vi "FFOvl.vi"(1 "Drv":u32=1) -> (0 "FFOvl":u8)   [LabVIEW 2017]
uses:
  ESLSCDLL.dll
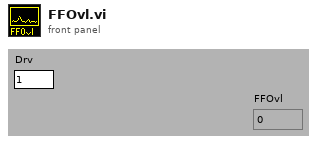
[diagram p1: front panel]
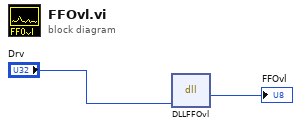
[diagram p0: block diagram]
diagram:
  n1 = dll-call lib="C:/ENTW/PCIE/64bit/lv64/lv64/board.vis/ESLSCDLL.dll" fn="DLLFFOvl"("drv"="Drv") -> ("Rückgabetyp"=→"FFOvl":u8)  [unwired: 4 in, 2 out]
